vi "TurnOffDeviceByFiveClockingHiSpeedDevice.vi"(0 "Handle":u32, 1 "error in (no error)":errorcluster) -> (2 "Handle":u32, 3 "Result":u32, 4 "error out":errorcluster)   [LabVIEW 2010]
uses:
  FTCSPI.dll
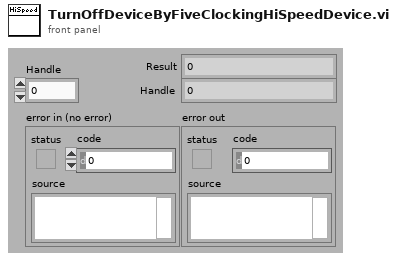
[diagram p1: front panel]
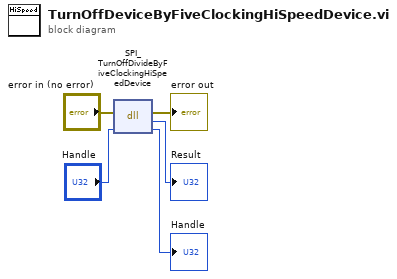
[diagram p0: block diagram]
diagram:
  n1 = dll-call lib="C:/Users/Administrator/Documents/GitHub/labview/FPGA/FTCSPI.dll" fn="SPI_TurnOffDivideByFiveClockingHiSpeedDevice"(error in="error in (no error)", "handle"="Handle") -> (error out=→"error out":errorcluster, "return type"=→"Result":u32, "handle"=→"Handle":u32)  [unwired: 2 in, 1 out]
